vi "processcmd.vi"(0 "VISA Refnum in":refnum<visa-resource-name>, 5 "write buffer":string, 11 "error in (no error)":errorcluster) -> (4 "VISA Refnum out":refnum<visa-resource-name>, 6 "read buffer":string, 15 "error out":errorcluster)   [LabVIEW 2020]
uses:
  haltnow.vi
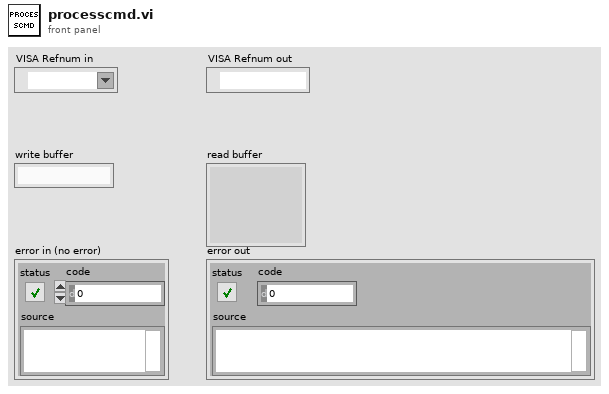
[diagram p1: front panel]
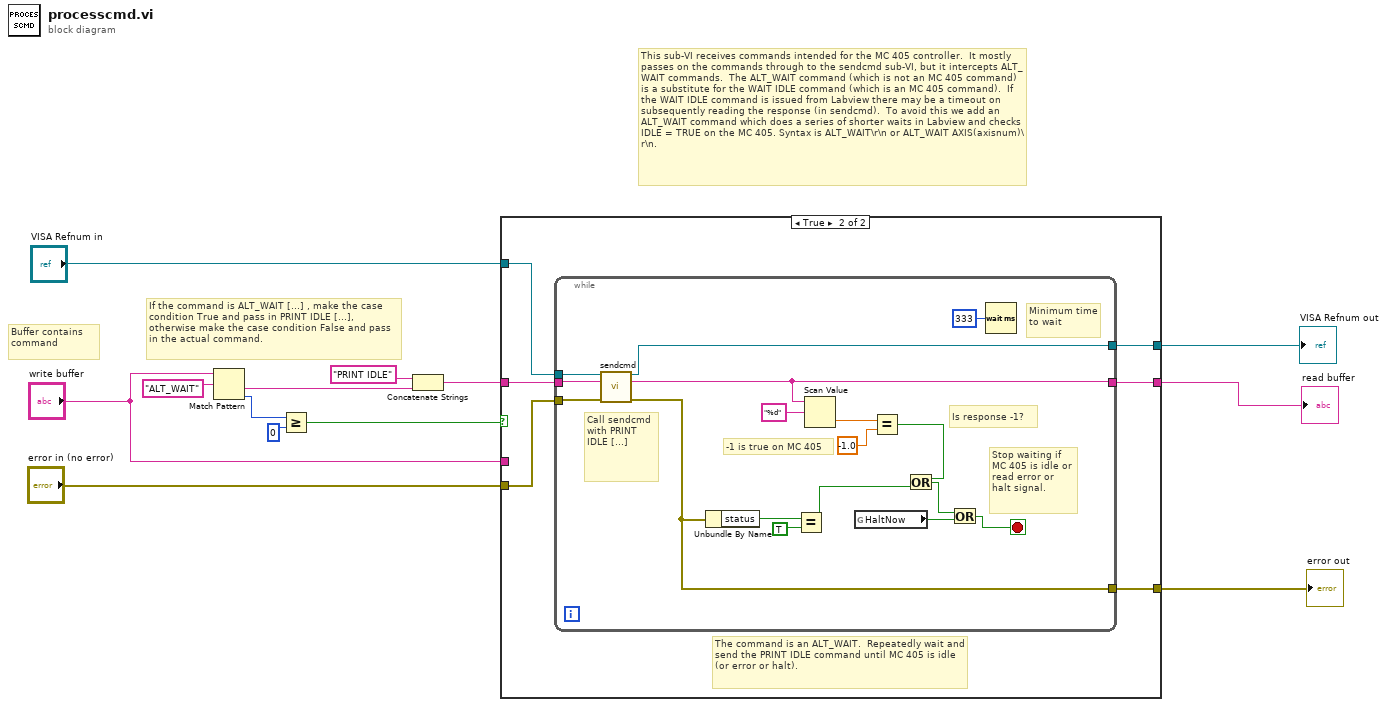
[diagram p0: block diagram]
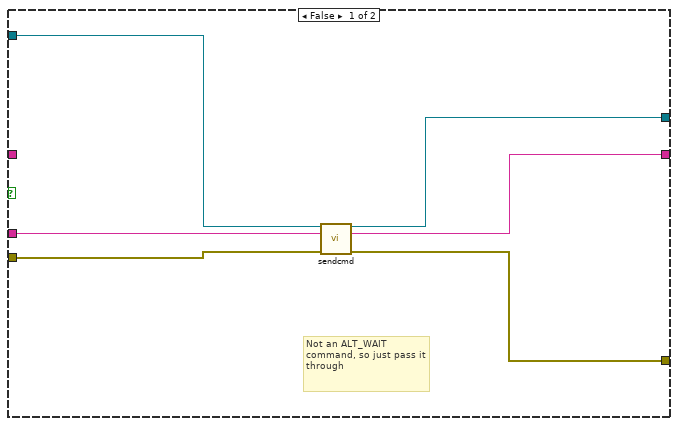
[diagram p2: hidden frame]
diagram:
  # "Buffer contains command"
  # "If the command is ALT_WAIT [...] , make the case condition True and pass in PRINT IDLE [...], otherwise make the case condition False and pass in the actual command."
  # "This sub-VI receives commands intended for the MC 405 controller.  It mostly passes on the commands through to the sendcmd sub-VI, but it intercepts ALT_WAIT commands.  The ALT_WAIT command (which is not an MC 405 command) is a substitute for the WAIT IDLE command (which is an MC 405 command).  If the WAIT IDLE command is issued from Labview there may be a timeout on subsequently reading the response (in sendcmd).  To avoid this we add an ALT_WAIT command which does a series of shorter waits in Labview and checks IDLE = TRUE on the MC 405. Syntax is ALT_WAIT\\r\\n or ALT_WAIT AXIS(axisnum)\\r\\n."
  n1 = Match Pattern(string="write buffer", regular expression="ALT_WAIT") -> (after substring=w12:string, offset past match=w10:i32)  [unwired: 1 in, 2 out]
  n2 = Greater Or Equal?(x=w10, y=0) -> (x >= y?=w8:bool)
  n3 = Concatenate Strings("PRINT IDLE" ("string"), w12) -> (w7:string)
  n4 = case shown="True" w8 {
    tunnel: w7 -> [_ w25]
    tunnel: "VISA Refnum in" -> [w19 w24]
    tunnel: "error in (no error)" -> [w18 w23]
    tunnel: [w17 w22] -> w4
    tunnel: [w16 w21] -> w3
    tunnel: [w15 w20] -> w2
    tunnel: "write buffer" -> [w14 _]
    frame False {
      # "Not an ALT_WAIT command, so just pass it through"
      n5 = call "sendcmd.vi"("VISA Refnum in"=w19, "write buffer"=w14, "error in (no error)"=w18) -> ("VISA Refnum out"=w17:refnum<visa-resource-name>, "read buffer"=w15:string, "error out"=w16:errorcluster)  [unwired: 10 in]
    }
    frame True {
      # "The command is an ALT_WAIT.  Repeatedly wait and send the PRINT IDLE command until MC 405 is idle (or error or halt)."
      n6 = while {
        tunnel: w25 -> [w42]
        tunnel: w24 -> [w41]
        tunnel: w23 -> [w40]
        tunnel: [w39] -> w22
        tunnel: [w33] -> w21
        tunnel: [w35] -> w20
        stop <- w28 stop-if-true
        # "Stop waiting if MC 405 is idle or read error or halt signal."
        # "Is response -1?"
        # "Call sendcmd with PRINT IDLE [...]"
        # "Minimum time to wait"
        # "-1 is true on MC 405"
        n7 = call "sendcmd.vi"("VISA Refnum in"=w41, "write buffer"=w42, "error in (no error)"=w40) -> ("VISA Refnum out"=w39:refnum<visa-resource-name>, "read buffer"=w35:string, "error out"=w33:errorcluster)  [unwired: 10 in]
        n8 = Unbundle By Name(w33) -> ("status"=w32:bool)
        n9 = Equal?(x=w32, y=TRUE) -> (x = y?=w30:bool)
        n10 = Scan Value(string=w35, format string="%d") -> (value=w37:dbl)  [unwired: 1 in, 1 out]
        n11 = global read "haltnow.vi" "HaltNow"() -> (w26:bool)
        n12 = Equal?(x=w37, y=-1.0) -> (x = y?=w29:bool)
        n13 = Or(x=w29, y=w30) -> (x .or. y?=w27:bool)
        n14 = Or(x=w27, y=w26) -> (x .or. y?=w28:bool)
        n15 = Wait (ms)(milliseconds to wait=u32 333) -> ()  [unwired: 1 out]
      }
    }
  }
  "read buffer" <- w2
  "error out" <- w3
  "VISA Refnum out" <- w4
